vi "getType.vi"(8 "error in (no error)":errorcluster, 11 "Structure In":refnum<class "Structure.lvclass">) -> (0 "error out":errorcluster, 2 "type":refnum<vi>, 3 "Structure Out":refnum<class "Structure.lvclass">)   [LabVIEW 2023, in "TLC_Scripto.lvlib" / "Structure.lvclass"]
uses:
  Structure.lvclass
  Structure.lvclass/Structure.ctl
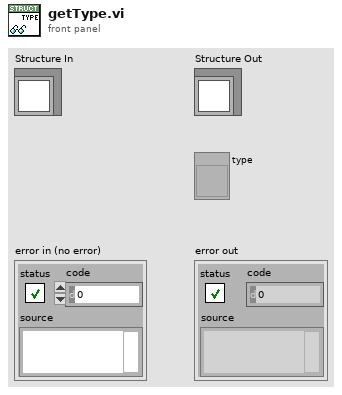
[diagram p1: front panel]
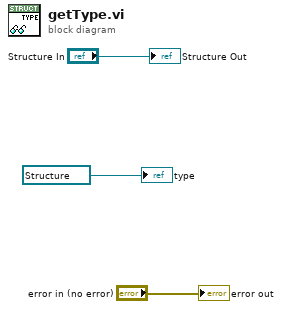
[diagram p0: block diagram]
diagram:
  "error out" <- "error in (no error)"
  "Structure Out" <- "Structure In"
  "type" <- refnum<vi> refnum ("type")
